vi "GBV_Ref.vi"() -> ()   [LabVIEW 2019]
panel:
  out "Stop":bool
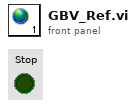
[diagram p1: front panel]
diagram:
